vi "Trigger.vi"(8 "error in (no error)":errorcluster, 11 "COGNEX IP:PORT(CMD)":string="192.168.0.30:23") -> (0 "error out":errorcluster, 1 "密碼":string, 2 "等待指令":string, 3 "Success":bool, 4 "及時":string, 5 "指令結果":string)   [LabVIEW 2019, in "Kolmogan Library 1.lvlib"]
uses:
  Kolmogan Library 1.lvlib
  <vilib>/regexp/Match Regular Expression.xnode
panel:
  out "x-y":dbl
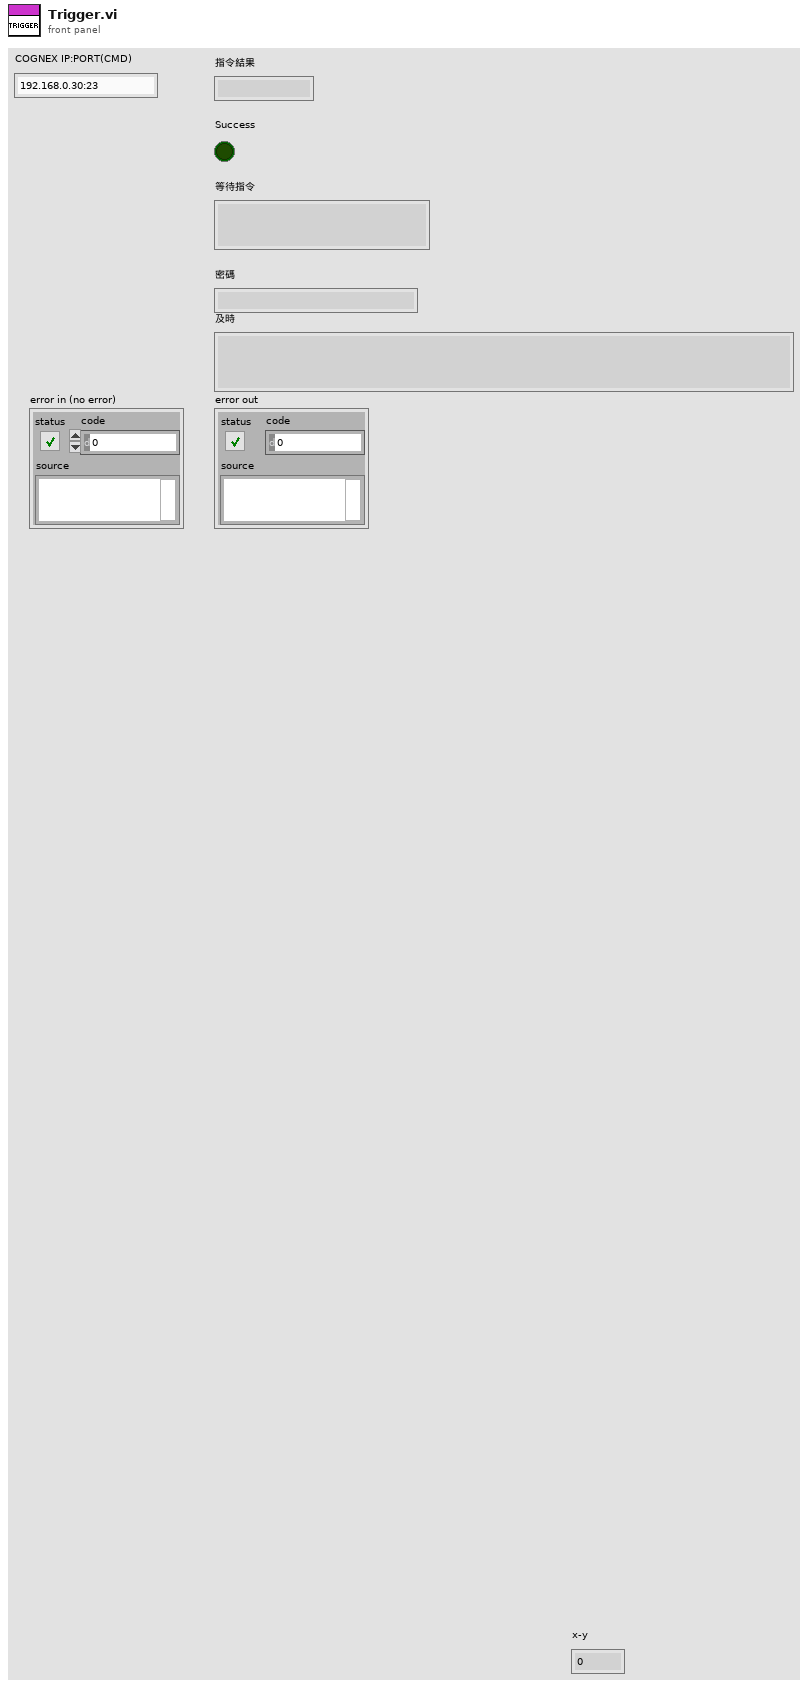
[diagram p1: front panel]
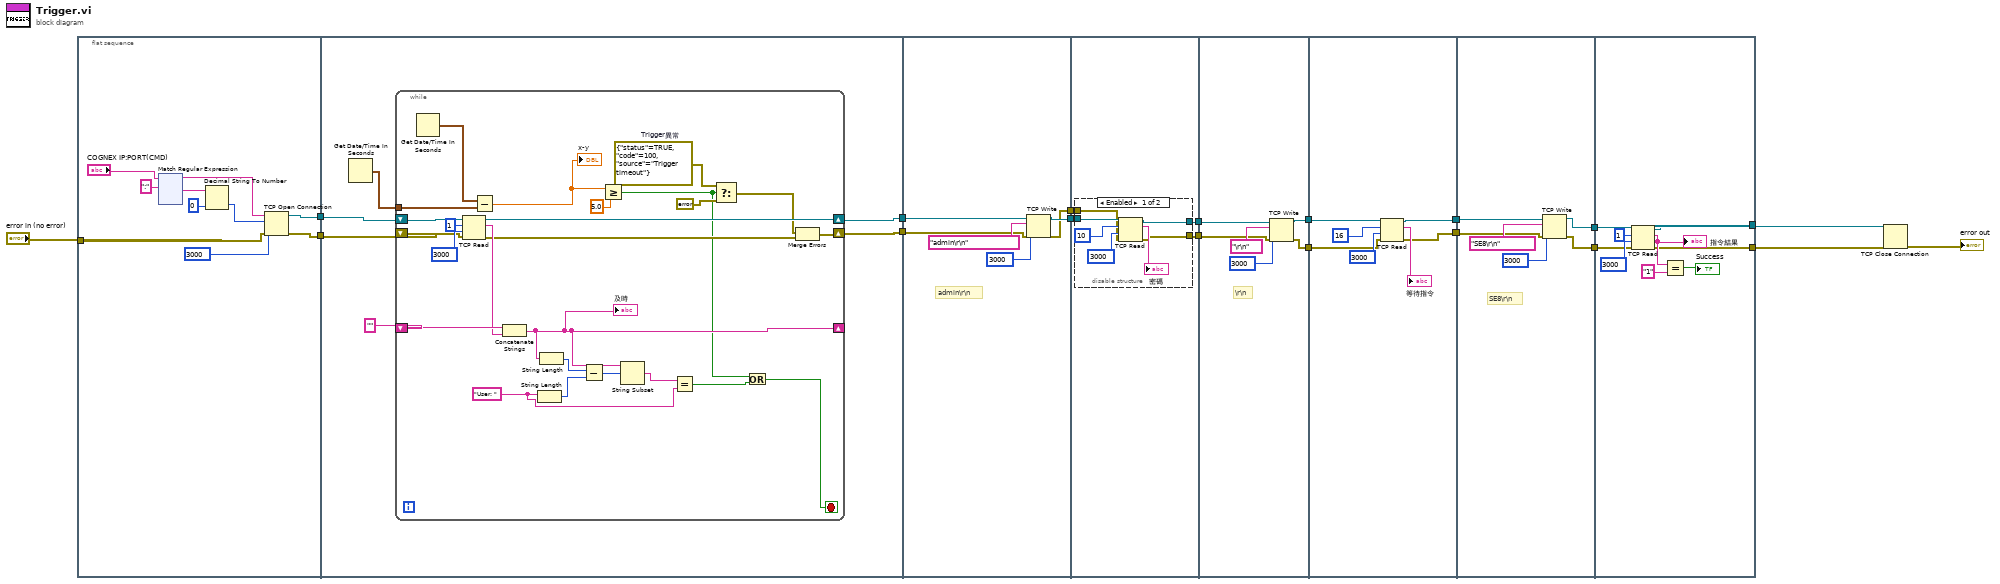
[diagram p0: block diagram]
diagram:
  n1 = flat-sequence {
    tunnel: [w27] -> w2
    tunnel: [w26] -> w1
    tunnel: "error in (no error)" -> [w25]
    tunnel: w2 -> [w148]
    tunnel: [w147] -> w18
    tunnel: w1 -> [w146]
    tunnel: [w145] -> w17
    tunnel: w18 -> [w179]
    tunnel: [w176] -> w16
    tunnel: w17 -> [w175]
    tunnel: [w174] -> w15
    tunnel: w16 -> [w183]
    tunnel: [w182] -> w14
    tunnel: w15 -> [w181]
    tunnel: [w180] -> w13
    tunnel: w14 -> [w195]
    tunnel: [w194] -> w12
    tunnel: w13 -> [w193]
    tunnel: [w192] -> w11
    tunnel: w12 -> [w202]
    tunnel: [w200] -> w10
    tunnel: w11 -> [w199]
    tunnel: [w198] -> w9
    tunnel: w10 -> [w208]
    tunnel: [w207] -> w8
    tunnel: w9 -> [w206]
    tunnel: [w205] -> w7
    tunnel: w8 -> [w217]
    tunnel: w7 -> [w213]
    tunnel: [w212] -> w3
    tunnel: [w211] -> w4
    frame #0 {
      n2 = xnode "Match Regular Expression"("input string"="COGNEX IP:PORT(CMD)", "regular expression"=":") -> ("before match"=w20:string, "after match"=w23:string)  [unwired: 4 in, 3 out]
      n3 = Decimal String To Number(string=w23, default (0L)=u16 0 ("default (0 I32)")) -> (number=w19:u16)  [unwired: 1 in, 1 out]
      n4 = TCP Open Connection(address=w20, remote port or service name=w19, timeout ms (60000)=3000, error in (no error)=w25) -> (connection ID=w27:refnum<k5>, error out=w26:errorcluster)  [unwired: 1 in]
    }
    frame #1 {
      n5 = Get Date/Time In Seconds() -> (seconds since 1Jan1904=w143:timestamp)
      n6 = while {
        shift-right: [w172] -> w147
        shift-left: w148 -> [w173]
        shift-right: [w154] -> w145
        shift-left: w146 -> [w169]
        shift-right: [w161] -> _
        shift-left: "" ("string") -> [w168]
        tunnel: w143 -> [w155]
        stop <- w149 stop-if-true
        w157 = errorcluster {"status"=TRUE, "code"=100, "source"="Trigger timeout"}  # Trigger異常
        w162 = "User: "
        n7 = Get Date/Time In Seconds() -> (seconds since 1Jan1904=w160:timestamp)
        n8 = TCP Read(connection ID=w173, bytes to read=1, error in (no error)=w169, 9:3000 ("timeout ms (25000)")) -> (connection ID out=w172:refnum<k5>, data out=w167:string, error out=w152:errorcluster)  [unwired: 1 in]
        n9 = Subtract(x=w160, y=w155) -> (x-y=w159:dbl)
        "x-y" <- w159
        n10 = Concatenate Strings(w168, w167) -> (w161:string)
        "及時" <- w161
        n11 = String Length(string=w162) -> (length=w165:i32)
        n12 = String Length(string=w161) -> (length=w166:i32)
        n13 = Subtract(x=w166, y=w165) -> (x-y=w164:i32)
        n14 = Greater Or Equal?(x=w159, y=5.0) -> (x >= y?=w150:bool)
        n15 = String Subset(string=w161, offset (0)=w164) -> (substring=w163:string)  [unwired: 1 in]
        n16 = Equal?(x=w163, y=w162) -> (x = y?=w151:bool)
        n17 = Select(t=w157, s=w150, f=errorcluster {"status"=FALSE, "code"=0, "source"=""} ("error out")) -> (s? t:f=w153:errorcluster)
        n18 = Or(x=w150, y=w151) -> (x .or. y?=w149:bool)
        n19 = Merge Errors(w153, w152) -> (w154:errorcluster)
      }
    }
    frame #2 {
      # "admin\\r\\n"
      n20 = TCP Write(connection ID=w179, data in="admin\r\n", error in (no error)=w175, 9:3000 ("timeout ms (25000)")) -> (connection ID out=w176:refnum<k5>, error out=w174:errorcluster)  [unwired: 1 out]
    }
    frame #3 {
      n21 = disable-structure shown="Enabled" {
        disable-tunnel: w183 -> [w188 w191]
        disable-tunnel: [w186 w191] -> w182
        disable-tunnel: w181 -> [w185 _]
        disable-tunnel: [w184 _] -> w180
        frame Enabled {
          n22 = TCP Read(connection ID=w188, bytes to read=10, error in (no error)=w185, 9:3000 ("timeout ms (25000)")) -> (connection ID out=w186:refnum<k5>, data out=→"密碼":string, error out=w184:errorcluster)  [unwired: 1 in]
        }
        frame Disabled {
        }
      }
    }
    frame #4 {
      # "\\r\\n"
      n23 = TCP Write(connection ID=w195, data in="\r\n", error in (no error)=w193, 9:3000 ("timeout ms (25000)")) -> (connection ID out=w194:refnum<k5>, error out=w192:errorcluster)  [unwired: 1 out]
    }
    frame #5 {
      n24 = TCP Read(connection ID=w202, bytes to read=16, error in (no error)=w199, 9:3000 ("timeout ms (25000)")) -> (connection ID out=w200:refnum<k5>, data out=→"等待指令":string, error out=w198:errorcluster)  [unwired: 1 in]
    }
    frame #6 {
      # "SE8\\r\\n"
      n25 = TCP Write(connection ID=w208, data in="SE8\r\n", error in (no error)=w206, 9:3000 ("timeout ms (25000)")) -> (connection ID out=w207:refnum<k5>, error out=w205:errorcluster)  [unwired: 1 out]
    }
    frame #7 {
      n26 = TCP Read(connection ID=w217, bytes to read=1, error in (no error)=w213, 9:3000 ("timeout ms (25000)")) -> (connection ID out=w211:refnum<k5>, data out=w216:string, error out=w212:errorcluster)  [unwired: 1 in]
      "指令結果" <- w216
      n27 = Equal?(x=w216, y="1") -> (x = y?=→"Success":bool)
    }
  }
  n28 = TCP Close Connection(connection ID=w4, error in (no error)=w3) -> (error out=→"error out":errorcluster)  [unwired: 1 in, 1 out]
